vi "OldCVTSetInlining.vi"(11 "inline?":bool) -> ()   [LabVIEW 2012, in "UnitTests.lvlib"]
uses:
  UnitTests.lvlib
panel:
  out "error out":errorcluster
  in  "error in":errorcluster
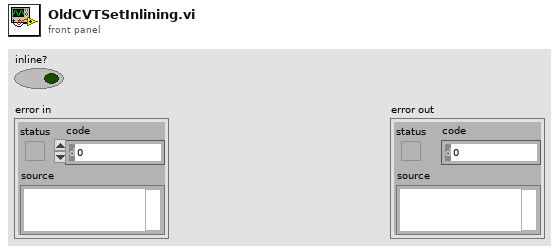
[diagram p1: front panel]
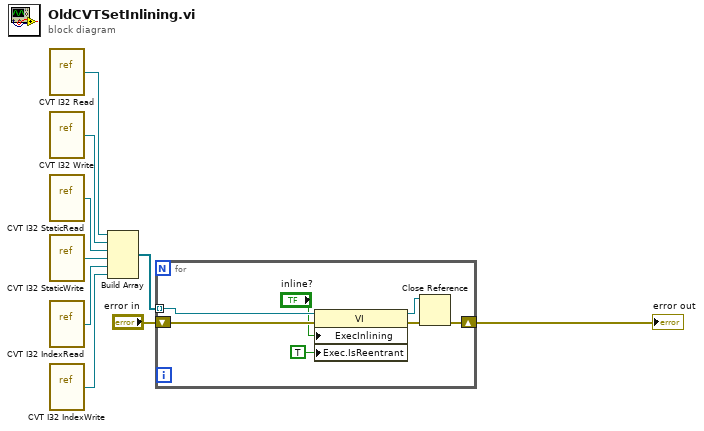
[diagram p0: block diagram]
diagram:
  n1 = vi-ref <userlib>:"CVT I32 Read.vi"() -> (w9:refnum<vi>)
  n2 = vi-ref <userlib>:"CVT I32 Write.vi"() -> (w8:refnum<vi>)
  n3 = vi-ref <userlib>:"CVT I32 StaticRead.vi"() -> (w7:refnum<vi>)
  n4 = vi-ref <userlib>:"CVT I32 StaticWrite.vi"() -> (w6:refnum<vi>)
  n5 = vi-ref <userlib>:"CVT I32 IndexRead.vi"() -> (w5:refnum<vi>)
  n6 = vi-ref <userlib>:"CVT I32 IndexWrite.vi"() -> (w4:refnum<vi>)
  n7 = Build Array(w9, w8, w7, w6, w5, w4) -> (w1:refnum<vi>[])
  n8 = for {
    tunnel: w1 -> [w16] mode=indexing
    shift-right: [w14] -> w2
    shift-left: "error in" -> [w15]
    n9 = property class="VI"(reference=w16, error in=w15, "ExecInlining"="inline?", "Exec.IsReentrant"=TRUE ("Execution:Is Reentrant")) -> (reference out=w13:refnum<vi>, error out=w12:errorcluster)
    n10 = Close Reference(reference=w13, error in (no error)=w12) -> (error out=w14:errorcluster)
  }
  "error out" <- w2
